vi "加标模块单控对话框.vi"(11 "标题":string="加标模块") -> ()   [LabVIEW 2016, in "质控单元.lvlib"]
uses:
  <vilib>/Utility/miscctls.llb/LVPointTypeDef.ctl
panel:
  in  "定位泵":bool
  in  "进样到液位":bool
  in  "排液":bool
  in  "退出":bool
  in  "柱塞泵":bool
  in  "排液":bool
  in  "搅拌":bool
  in  "进样调速":bool
  in  "进样":bool
  in  "停止":bool
  in  "加标启动":bool
  # "手动控制"
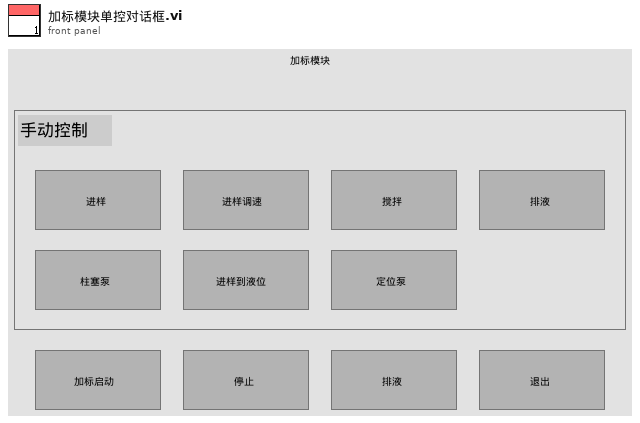
[diagram p1: front panel]
types:
  T1 = typedef "LVPointTypeDef.ctl" = cluster{"Horizontal":i16, "Vertical":i16}
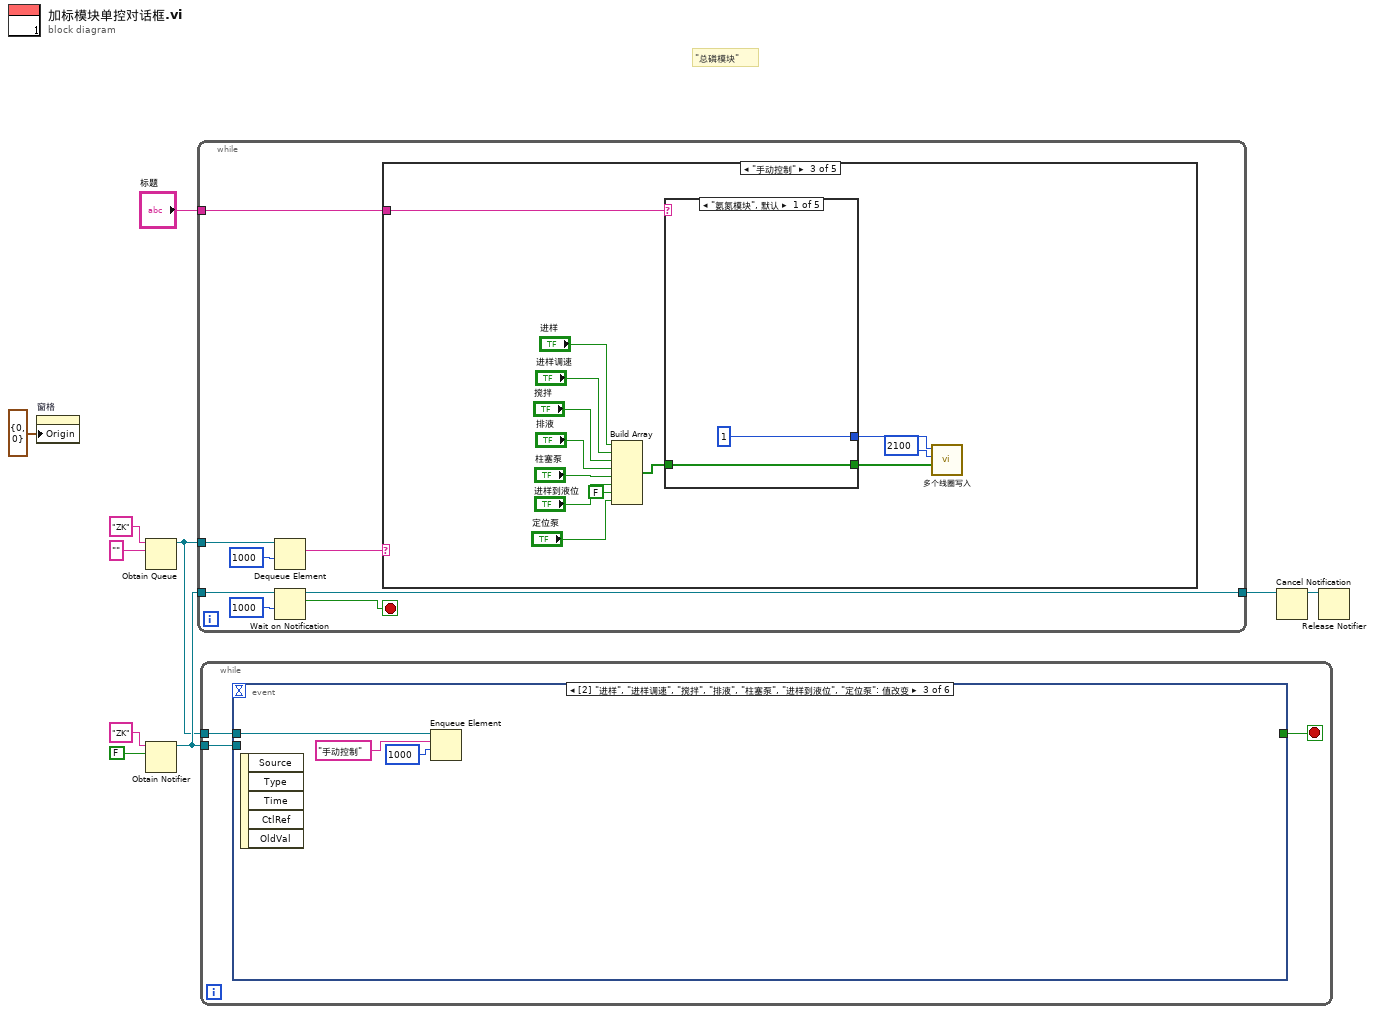
[diagram p0: block diagram]
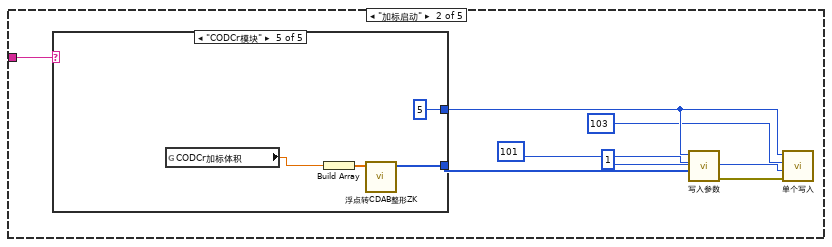
[diagram p3: hidden frame]
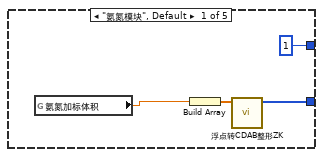
[diagram p4: hidden frame]
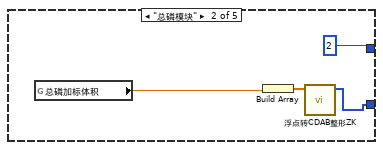
[diagram p5: hidden frame]
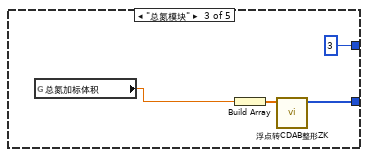
[diagram p6: hidden frame]
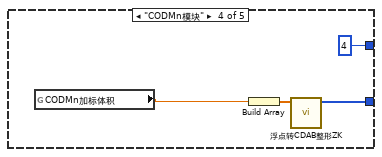
[diagram p7: hidden frame]
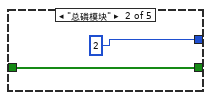
[diagram p8: hidden frame]
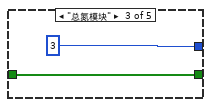
[diagram p9: hidden frame]
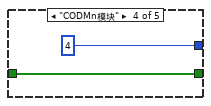
[diagram p10: hidden frame]
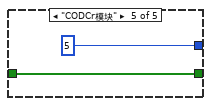
[diagram p11: hidden frame]
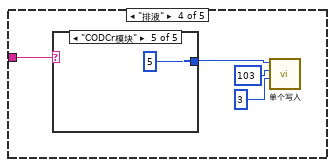
[diagram p12: hidden frame]
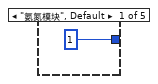
[diagram p13: hidden frame]
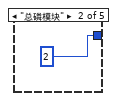
[diagram p14: hidden frame]
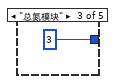
[diagram p15: hidden frame]
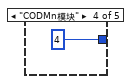
[diagram p16: hidden frame]
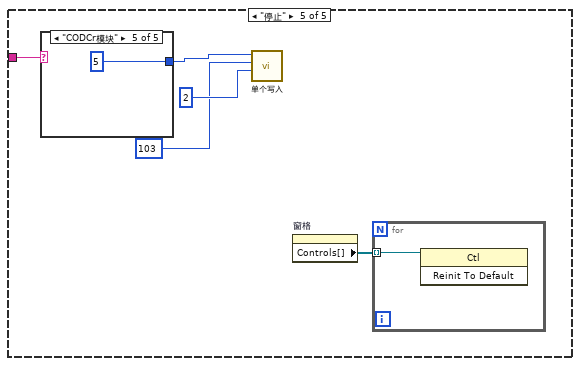
[diagram p17: hidden frame]
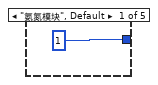
[diagram p18: hidden frame]
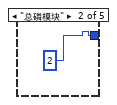
[diagram p19: hidden frame]
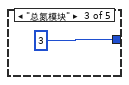
[diagram p20: hidden frame]
diagram:
  # "\"总磷模块\""
  n1 = property on="窗格" class="Pane"("Origin"=T1 {"Horizontal"=0, "Vertical"=0} ("原点")) -> ()  [unwired: 2 in, 2 out]
  n2 = Obtain Queue(name (unnamed)="ZK" ("名称（未命名）"), element data type="" ("名称（未命名）")) -> (queue out=w3:refnum<queue>)  [unwired: 3 in, 2 out]
  n3 = Obtain Notifier(name (unnamed)="ZK" ("名称（未命名）"), notification data type=FALSE) -> (notifier out=w8:refnum<notifier>)  [unwired: 2 in, 2 out]
  n4 = while {
    tunnel: w8 -> [w18]
    tunnel: [w16] -> w7
    tunnel: w3 -> [w15]
    tunnel: "标题" -> [w11]
    stop <- w17 stop-if-true
    n5 = Dequeue Element(queue=w15, timeout in ms (-1)=1000 ("超时毫秒(-1)")) -> (element=w14:string)  [unwired: 1 in, 3 out]
    n6 = Wait on Notification(notifier=w18, timeout in ms (-1)=1000 ("超时毫秒(-1)")) -> (notifier out=w16:refnum<notifier>, notification=w17:bool)  [unwired: 2 in, 2 out]
    n7 = case shown="\"手动控制\"" w14 {
      tunnel: w11 -> [_ w19 w48 w69 w79]
      frame Default {
      }
      frame "加标启动" {
        n8 = case shown="\"CODCr模块\"" w19 {
          tunnel: [w28 w33 w36 w40 w44] -> w21
          tunnel: [u8 1 ("Slave ID") u8 2 ("Slave ID") u8 3 ("Slave ID") u8 4 ("Slave ID") u8 5 ("Slave ID")] -> w25
          frame "氨氮模块", Default {
            n9 = global read "加标回收状态全局变量.vi" "氨氮加标体积"() -> (w26:dbl)
            n10 = Build Array(w26) -> (w29:dbl[])
            n11 = call "浮点转CDAB整形ZK.vi"("浮点数"=w29) -> ("CDAB整形输出"=w28:u16[])  [unwired: 10 in]
          }
          frame "总磷模块" {
            n12 = global read "加标回收状态全局变量.vi" "总磷加标体积"() -> (w31:dbl)
            n13 = Build Array(w31) -> (w30:dbl[])
            n14 = call "浮点转CDAB整形ZK.vi"("浮点数"=w30) -> ("CDAB整形输出"=w33:u16[])  [unwired: 10 in]
          }
          frame "总氮模块" {
            n15 = global read "加标回收状态全局变量.vi" "总氮加标体积"() -> (w34:dbl)
            n16 = Build Array(w34) -> (w37:dbl[])
            n17 = call "浮点转CDAB整形ZK.vi"("浮点数"=w37) -> ("CDAB整形输出"=w36:u16[])  [unwired: 10 in]
          }
          frame "CODMn模块" {
            n18 = global read "加标回收状态全局变量.vi" "CODMn加标体积"() -> (w38:dbl)
            n19 = Build Array(w38) -> (w41:dbl[])
            n20 = call "浮点转CDAB整形ZK.vi"("浮点数"=w41) -> ("CDAB整形输出"=w40:u16[])  [unwired: 10 in]
          }
          frame "CODCr模块" {
            n21 = global read "加标回收状态全局变量.vi" "CODCr加标体积"() -> (w42:dbl)
            n22 = Build Array(w42) -> (w45:dbl[])
            n23 = call "浮点转CDAB整形ZK.vi"("浮点数"=w45) -> ("CDAB整形输出"=w44:u16[])  [unwired: 10 in]
          }
        }
        n24 = call "写入参数.vi"("values"=w21, "starting address"=u16 101, "Slave ID"=w25) -> ("error out"=w20:errorcluster)  [unwired: 8 in]
        n25 = call "单个写入.vi"("Error in"=w20, "value"=u16 1, "address"=u16 103, "Slave ID"=w25) -> ()  [unwired: 7 in, 1 out]
      }
      frame "手动控制" {
        n26 = Build Array("进样", "进样调速", "搅拌", "排液", "柱塞泵", "进样到液位", FALSE ("元素"), "定位泵") -> (w54:bool[])
        n27 = case shown="\"氨氮模块\", 默认" w48 {
          tunnel: w54 -> [w60 w62 w63 w66 w68]
          tunnel: [w60 w62 w63 w66 w68] -> w55
          tunnel: [u8 1 ("Slave ID") u8 2 ("Slave ID") u8 3 ("Slave ID") u8 4 ("Slave ID") u8 5 ("Slave ID")] -> w57
          frame "氨氮模块", Default {
          }
          frame "总磷模块" {
          }
          frame "总氮模块" {
          }
          frame "CODMn模块" {
          }
          frame "CODCr模块" {
          }
        }
        n28 = call "多个线圈写入.vi"("values"=w55, "starting address"=u16 2100, "Slave ID"=w57) -> ()  [unwired: 8 in, 1 out]
      }
      frame "排液" {
        n29 = case shown="\"CODCr模块\"" w69 {
          tunnel: [u8 1 ("Slave ID") u8 2 ("Slave ID") u8 3 ("Slave ID") u8 4 ("Slave ID") u8 5 ("Slave ID")] -> w70
          frame "氨氮模块", Default {
          }
          frame "总磷模块" {
          }
          frame "总氮模块" {
          }
          frame "CODMn模块" {
          }
          frame "CODCr模块" {
          }
        }
        n30 = call "单个写入.vi"("value"=u16 3, "address"=u16 103, "Slave ID"=w70) -> ()  [unwired: 8 in, 1 out]
      }
      frame "停止" {
        n31 = case shown="\"CODCr模块\"" w79 {
          tunnel: [u8 1 ("Slave ID") u8 2 ("Slave ID") u8 3 ("Slave ID") u8 4 ("Slave ID") u8 5 ("Slave ID")] -> w80
          frame "氨氮模块", Default {
          }
          frame "总磷模块" {
          }
          frame "总氮模块" {
          }
          frame "CODMn模块" {
          }
          frame "CODCr模块" {
          }
        }
        n32 = call "单个写入.vi"("value"=u16 2, "address"=u16 103, "Slave ID"=w80) -> ()  [unwired: 8 in, 1 out]
        n33 = property on="窗格" class="Pane"() -> ("Controls[]"=w78:refnum<vi>[])  [unwired: 2 in, 2 out]
        n34 = for {
          tunnel: w78 -> [w83] mode=indexing
          n35 = invoke class="Ctl" method="Reinit To Default"(reference=w83) -> ()  [unwired: 2 in, 3 out]
        }
      }
    }
  }
  n36 = while {
    tunnel: w8 -> [w90]
    tunnel: w3 -> [w89]
    stop <- w91 stop-if-true
    n37 = event shown="[2] \"进样\", \"进样调速\", \"搅拌\", \"排液\", \"柱塞泵\", \"进样到液位\", \"定位泵\": 值改变" {
      selector: _ -> [_ _ _ _ _ _]
      dyn-events: _ -> [_ _ _ _ _ _]
      timeout: _ -> [_ _ _ _ _ _]
      tunnel: [_ _ _ _ _ TRUE] -> w91
      tunnel: w90 -> [_ _ _ _ _ w107]
      tunnel: w89 -> [_ w94 w95 w98 w103 w106]
      event Timeout {
        n38 = event-data() -> ()  [unwired: 1 in, 3 out]
      }
      event "加标启动": Value Change {
        n39 = event-data() -> ()  [unwired: 1 in, 4 out]
        n40 = Enqueue Element(queue=w94, element="加标启动" ("元素"), timeout in ms (-1)=1000 ("超时毫秒(-1)")) -> ()  [unwired: 1 in, 3 out]
      }
      event "进样", "进样调速", "搅拌", "排液", "柱塞泵", "进样到液位", "定位泵": Value Change {
        n41 = event-data() -> ()  [unwired: 1 in, 5 out]
        n42 = Enqueue Element(queue=w95, element="手动控制" ("元素"), timeout in ms (-1)=1000 ("超时毫秒(-1)")) -> ()  [unwired: 1 in, 3 out]
      }
      event "排液": Value Change {
        n43 = event-data() -> ()  [unwired: 1 in, 6 out]
        n44 = Enqueue Element(queue=w98, element="排液" ("元素"), timeout in ms (-1)=1000 ("超时毫秒(-1)")) -> ()  [unwired: 1 in, 3 out]
      }
      event "停止": Value Change {
        n45 = event-data() -> ()  [unwired: 1 in, 5 out]
        n46 = Flush Queue(queue=w103) -> (queue out=w102:refnum<queue>)  [unwired: 1 in, 2 out]
        n47 = Enqueue Element(queue=w102, element="停止" ("元素"), timeout in ms (-1)=1000 ("超时毫秒(-1)")) -> ()  [unwired: 1 in, 3 out]
      }
      event "退出": Value Change; Panel Close {
        n48 = event-data() -> ()  [unwired: 1 in, 3 out]
        n49 = Send Notification(notification=TRUE ("通知"), notifier=w107) -> ()  [unwired: 1 in, 2 out]
        n50 = Flush Queue(queue=w106) -> (queue out=w105:refnum<queue>)  [unwired: 1 in, 2 out]
        n51 = Two Button Dialog(message="请确认是否退出，退出仪器将停止运行" ("消息"), 1:"N" ("F按钮名称（“取消”）"), 2:"Y" ("T按钮名称（“确定”）")) -> (T button?=w109:bool)
        n52 = case shown="真" w109 {
          tunnel: w105 -> [_ w114]
          frame False {
          }
          frame True {
            n53 = property on="窗格" class="Pane"() -> ("Controls[]"=w117:refnum<vi>[])  [unwired: 2 in, 2 out]
            n54 = Enqueue Element(queue=w114, element="停止" ("元素"), timeout in ms (-1)=1000 ("超时毫秒(-1)")) -> ()  [unwired: 1 in, 3 out]
            n55 = for {
              tunnel: w117 -> [w118] mode=indexing
              n56 = invoke class="Ctl" method="Reinit To Default"(reference=w118) -> ()  [unwired: 2 in, 3 out]
            }
          }
        }
      }
    }
  }
  n57 = Cancel Notification(0:w7) -> (8:w6:refnum<notifier>)  [unwired: 1 in, 2 out]
  n58 = Release Notifier(notifier=w6) -> ()  [unwired: 2 in, 3 out]
